vi "UI_KBB_Trig.vi"(8 "error in (no error)":errorcluster, 11 "UI_Actor in":refnum<class "UI_Actor.lvclass">) -> (0 "error out":errorcluster, 3 "UI_Actor out":refnum<class "UI_Actor.lvclass">)   [LabVIEW 2020, in "UI_Actor.lvlib" / "UI_Actor.lvclass"]
doc: "Ce VI déchenche un arrêt par le bas. \nL'acteur considéré s'auto-triggera un stop (standard) quand tous ses nested seront arretés."
uses:
  UI_Actor.lvclass
  D:/Projets/STEP AT/UI Actor/support/Actor Framework.lvlibp/1abvi3w/vi.lib/ActorFramework/Actor/Actor.lvclass
  UI_Actor.lvclass/UI_Actor.ctl
  support/Actor Framework.lvlibp/1abvi3w/vi.lib/ActorFramework/Message Enqueuer/Enqueue.vi
  UI_Actor Messages/UI_KBB_Trig Msg/UI_KBB_Trig Msg.lvclass
  support/Actor Framework.lvlibp/1abvi3w/vi.lib/ActorFramework/Actor/Actor.lvclass
  support/Actor Framework.lvlibp/1abvi3w/vi.lib/ActorFramework/Stop Msg/Stop Msg.lvclass
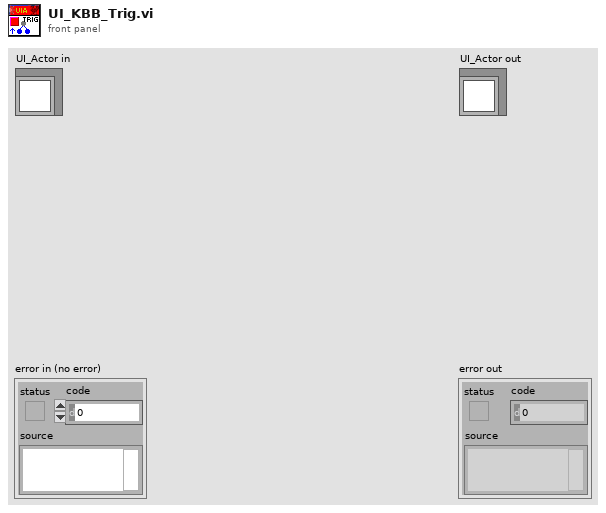
[diagram p1: front panel]
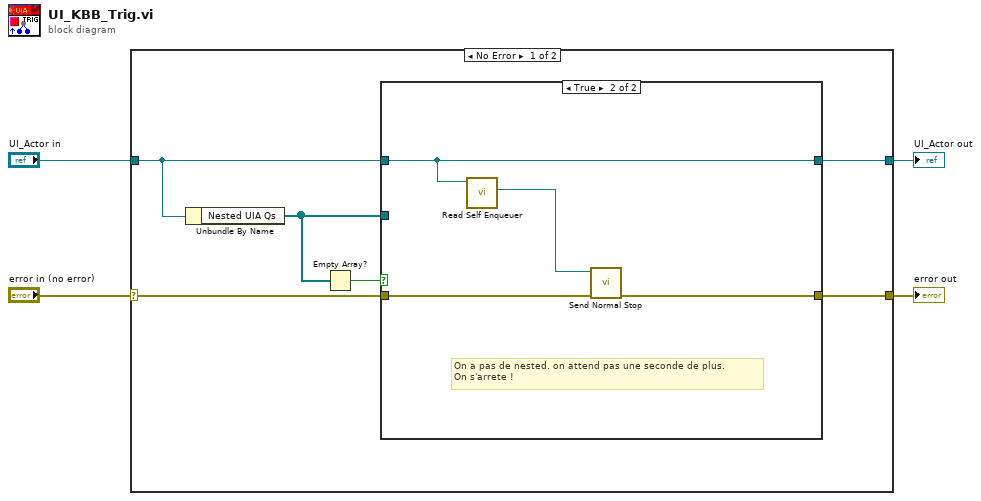
[diagram p0: block diagram]
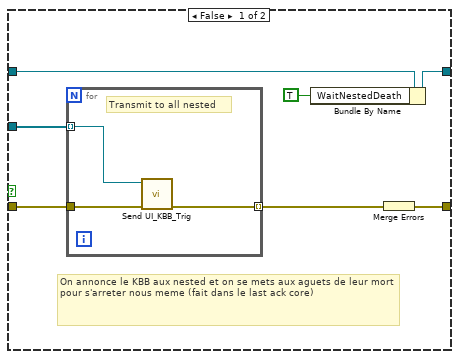
[diagram p2: hidden frame]
diagram:
  n1 = case shown="No Error" "error in (no error)" {
    selector: "error in (no error)" -> [w7 w26]
    tunnel: [w6 w26] -> w3
    tunnel: [w8 w25] -> w1
    tunnel: "UI_Actor in" -> [w9 w25]
    frame No Error {
      n2 = Unbundle By Name(w9) -> ("Nested UIA Qs"=w5:refnum<class "Message Enqueuer.lvclass">[])
      n3 = Empty Array?(array=w5) -> (empty?=w10:bool)
      n4 = case shown="True" w10 {
        tunnel: w9 -> [w17 w24]
        tunnel: [w14 w24] -> w8
        tunnel: w7 -> [w15 w22]
        tunnel: [w11 w21] -> w6
        tunnel: w5 -> [w16 _]
        frame False {
          # "On annonce le KBB aux nested et on se mets aux aguets de leur mort pour s'arreter nous meme (fait dans le last ack core)"
          n5 = for {
            tunnel: w16 -> [w18] mode=indexing
            tunnel: w15 -> [w20]
            tunnel: [w19] -> w12 mode=indexing
            # "Transmit to all nested"
            n6 = call "Send UI_KBB_Trig.vi"("error in (no error)"=w20, "Message Enqueuer"=w18) -> ("error out"=w19:errorcluster)  [unwired: 8 in, 1 out]
          }
          n7 = Bundle By Name(cluster=w17, "WaitNestedDeath"=TRUE) -> (w14:refnum<class "UI_Actor.lvclass">)
          n8 = Merge Errors(w12) -> (w11:errorcluster)
        }
        frame True {
          # "On a pas de nested. on attend pas une seconde de plus.\nOn s'arrete !"
          n9 = call "Read Self Enqueuer.vi"("Actor"=w24) -> ("Self Enqueuer"=w23:refnum<class "Message Enqueuer.lvclass">)  [unwired: 10 in]
          n10 = call "Send Normal Stop.vi"("error in (no error)"=w22, "Message Enqueuer"=w23) -> ("error out"=w21:errorcluster)  [unwired: 9 in]
        }
      }
    }
    frame Error {
    }
  }
  "error out" <- w3
  "UI_Actor out" <- w1
